vi "Sorting_Single_Frame_Displ_2.vi"(0 "(X,Y,dX,dY) IN":dbl[][](array[numeric]), 2 "error IN":errorcluster) -> (3 "Displ >1 Frame":dbl[][](array[numeric]), 4 "Displ =1 Frame":dbl[][](array[numeric]), 6 "error OUT":errorcluster)   [LabVIEW 2013]
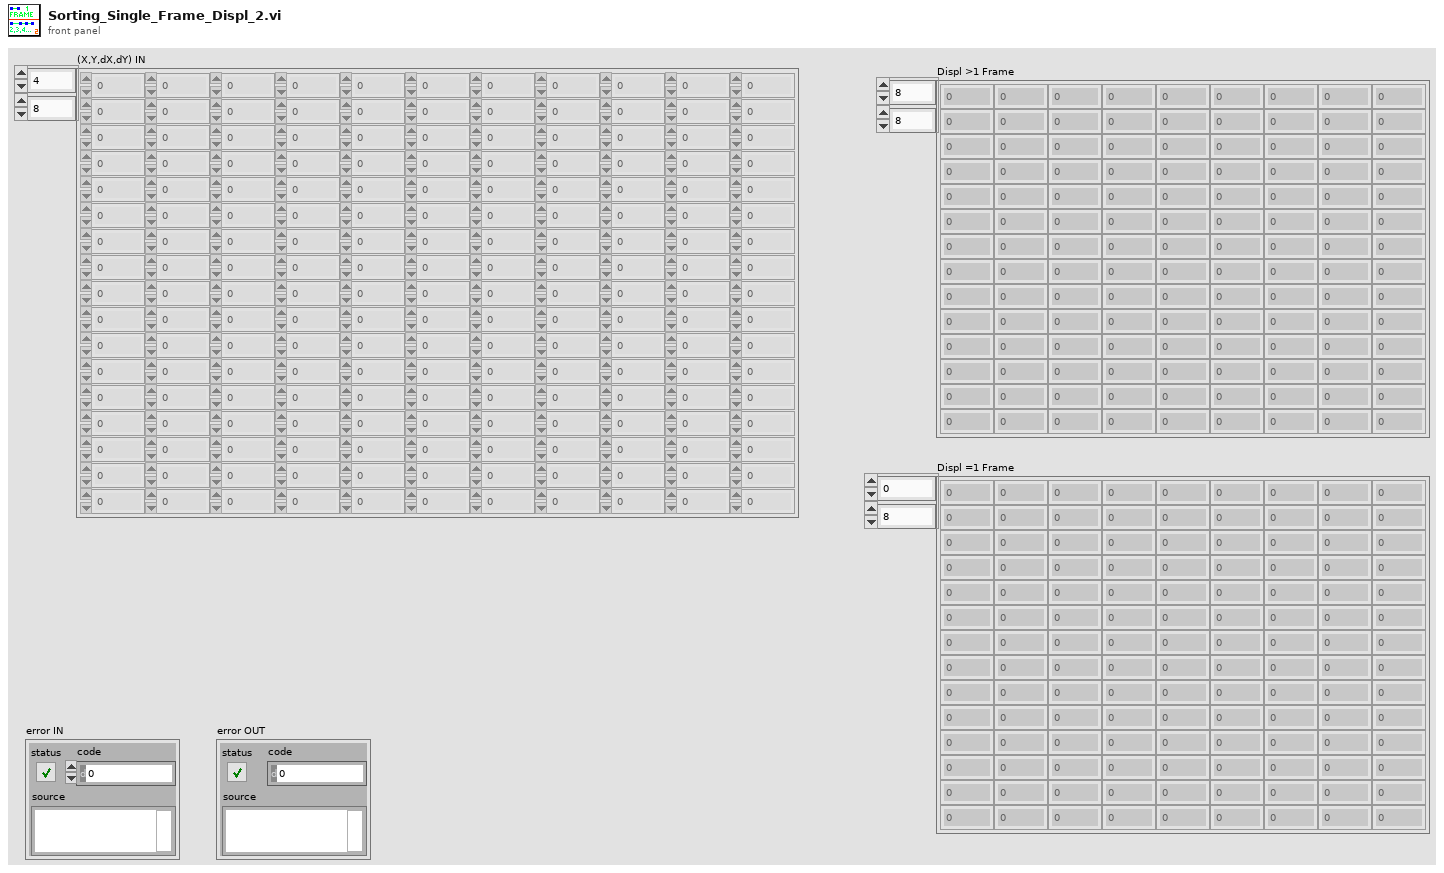
[diagram p1: front panel]
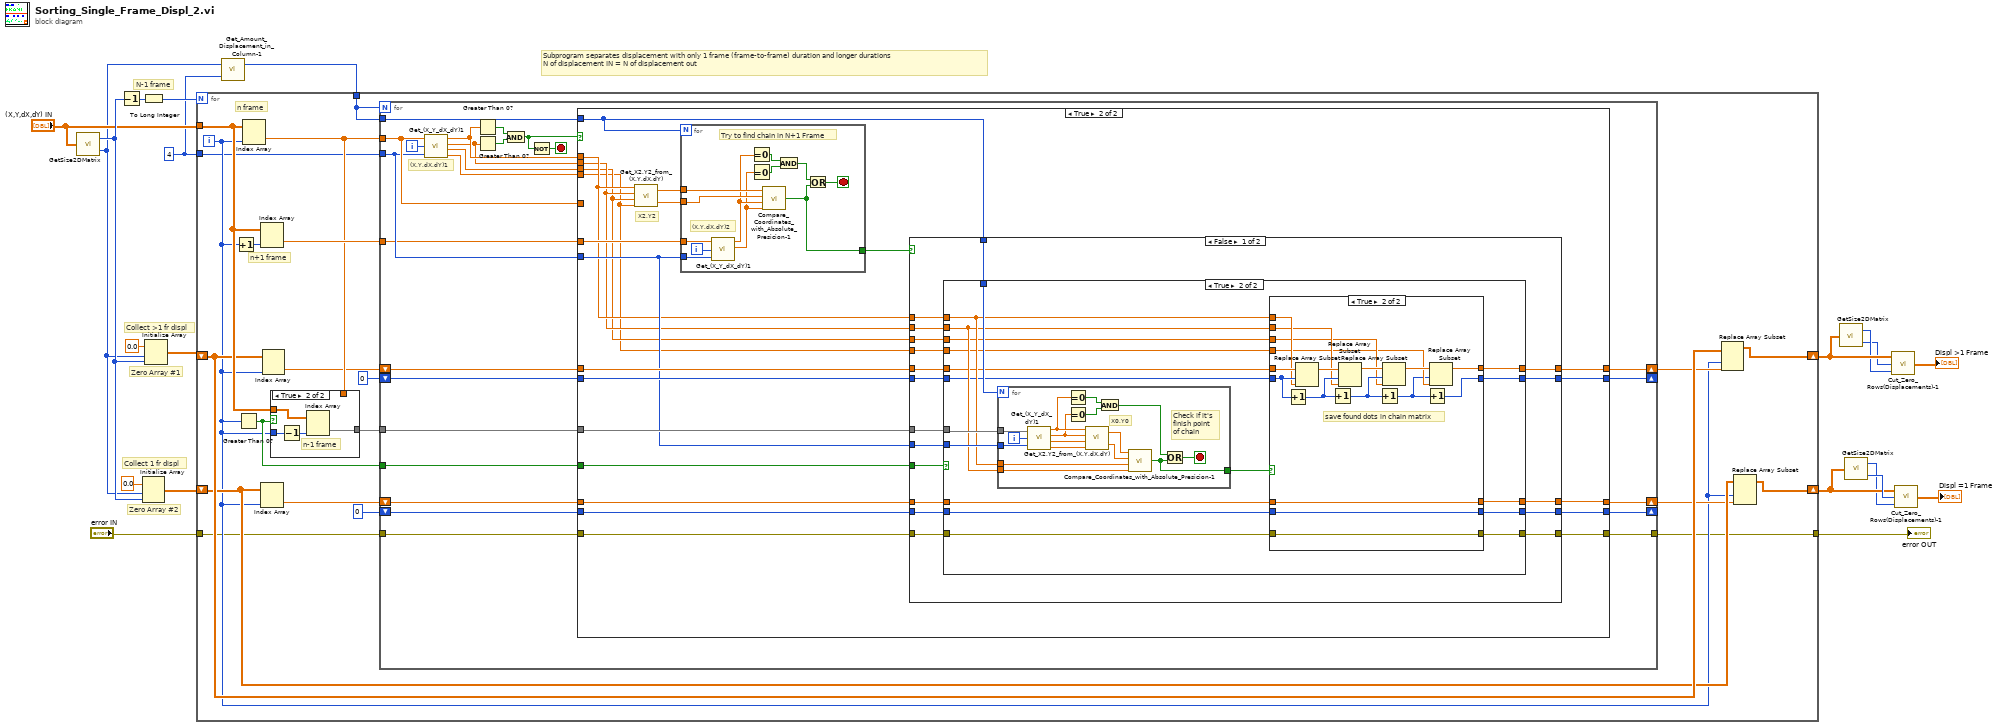
[diagram p0: block diagram]
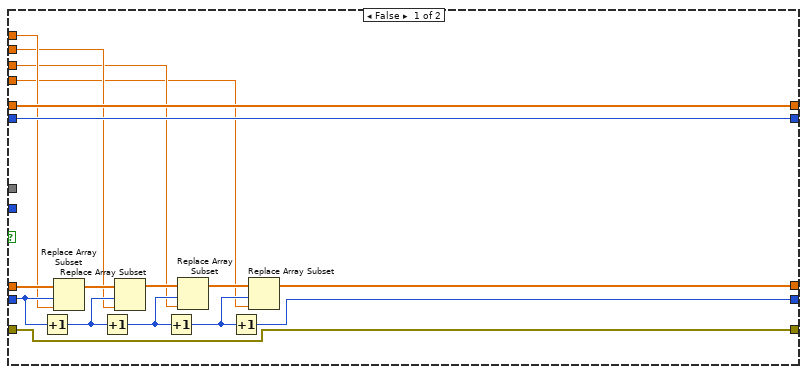
[diagram p4: hidden frame]
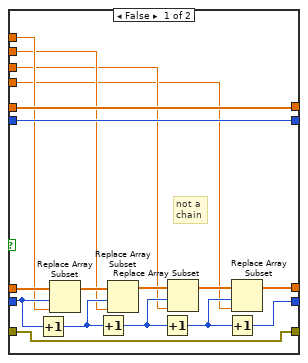
[diagram p5: hidden frame]
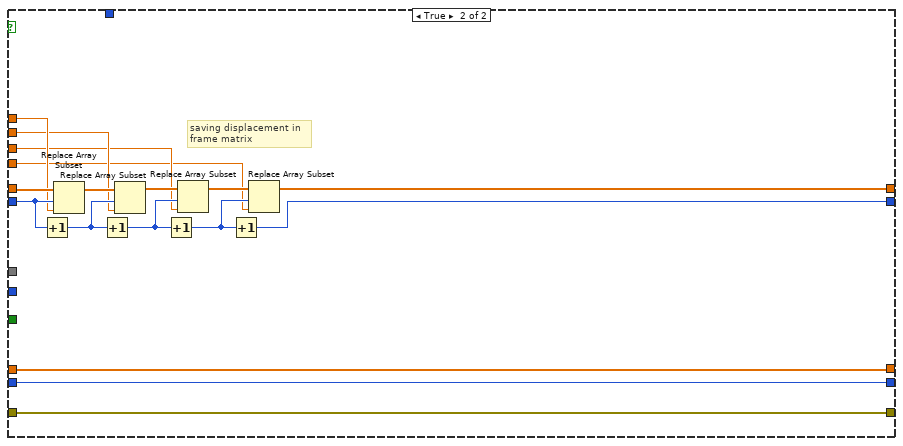
[diagram p6: hidden frame]
diagram:
  w2 = 4 ("y")
  # "Collect >1 fr displ"
  # "Collect 1 fr displ"
  # "Subprogram separates displacement with only 1 frame (frame-to-frame) duration and longer durations\nN of displacement IN = N of displacement out"
  # "Zero Array #2"
  # "Zero Array #1"
  # "N-1 frame"
  n1 = call "GetSize2DMatrix.vi"("Array IN (2D)"="(X,Y,dX,dY) IN") -> ("# Cols"=w16:i32, "# Rows"=w3:i32)
  n2 = Decrement(x=w16) -> (x-1=w21:i32)
  n3 = To Long Integer(number=w21) -> (32bit integer=w19:i32)
  n4 = Initialize Array(0.0 ("element"), w3, w16) -> (w15:dbl[][])
  n5 = Initialize Array(0.0 ("element"), w3, w16) -> (w18:dbl[][])
  n6 = call "Get_Amount_Displacement_in_Column-1.vi"("multiplier"=w2, "# Rows"=w3) -> ("Displ amount"=w1:i32)  [unwired: 1 out]
  n7 = for {
    N: w19 -> [_]
    shift-right: [w31] -> w13
    shift-left: w18 -> [w33]
    shift-right: [w27] -> w9
    shift-left: w15 -> [w29]
    tunnel: "(X,Y,dX,dY) IN" -> [w40]
    tunnel: "error IN" -> [w25]
    tunnel: [w24] -> w7
    tunnel: w2 -> [w23]
    tunnel: w1 -> [w22]
    i -> [w26]
    # "n+1 frame"
    # "n frame"
    n8 = Increment(x=w26) -> (x+1=w42:i32)
    n9 = Greater Than 0?(x=w26) -> (x > 0?=w37:bool)
    n10 = Index Array(array=w40, index (col)=w26) -> (element=w38:dbl[])  [unwired: 1 in]
    n11 = Index Array(array=w40, index (col)=w42) -> (element=w41:dbl[])  [unwired: 1 in]
    n12 = Index Array(array=w29, index (col)=w26) -> (element=w35:dbl[])  [unwired: 1 in]
    n13 = Index Array(array=w33, index (col)=w26) -> (element=w36:dbl[])  [unwired: 1 in]
    n14 = case shown="True" w37 {
      tunnel: w40 -> [_ w47]
      tunnel: w26 -> [_ w45]
      tunnel: [w43 w46] -> w39
      tunnel: w38 -> [w43 _]
      frame False {
      }
      frame True {
        # "n-1 frame"
        n15 = Decrement(x=w45) -> (x-1=w44:i32)
        n16 = Index Array(array=w47, index (col)=w44) -> (element=w46:dbl[])  [unwired: 1 in]
      }
    }
    n17 = for {
      N: w22 -> [_]
      tunnel: w41 -> [w62]
      tunnel: w23 -> [w67]
      tunnel: w22 -> [w69]
      tunnel: w38 -> [w68]
      tunnel: w39 -> [w54]
      tunnel: w37 -> [w59]
      shift-right: [w56] -> w32
      shift-left: w36 -> [w57]
      shift-right: [w50] -> w28
      shift-left: w35 -> [w53]
      shift-right: [w55] -> _
      shift-left: 0 -> [w58]
      shift-right: [w51] -> _
      shift-left: 0 -> [w52]
      tunnel: w25 -> [w49]
      tunnel: [w48] -> w24
      i -> [w72]
      stop <- w61 stop-if-true
      # "(X,Y,dX,dY)1"
      n18 = call "Get_(X_Y_dX_dY)1.vi"("(X,Y,dX,dY)"=w68, "index"=w72, "multiplier"=w67) -> ("X"=w66:dbl, "Y"=w65:dbl, "dX"=w64:dbl, "dY"=w63:dbl)
      n19 = Greater Than 0?(x=w66) -> (x > 0?=w71:bool)
      n20 = Greater Than 0?(x=w65) -> (x > 0?=w70:bool)
      n21 = And(x=w71, y=w70) -> (x .and. y?=w60:bool)
      n22 = Not(x=w60) -> (.not. x?=w61:bool)
      n23 = case shown="True" w60 {
        tunnel: w69 -> [_ w86]
        tunnel: w68 -> [_ _]
        tunnel: w67 -> [_ w87]
        tunnel: w66 -> [_ w83]
        tunnel: w65 -> [_ w80]
        tunnel: w64 -> [_ w79]
        tunnel: w63 -> [_ w78]
        tunnel: w62 -> [_ w99]
        tunnel: w59 -> [_ w95]
        tunnel: w58 -> [w76 w96]
        tunnel: w57 -> [w77 w97]
        tunnel: [w77 w90] -> w56
        tunnel: [w76 w89] -> w55
        tunnel: w54 -> [_ w88]
        tunnel: w53 -> [w75 w94]
        tunnel: w52 -> [w74 w93]
        tunnel: [w74 w91] -> w51
        tunnel: [w75 w92] -> w50
        tunnel: w49 -> [w73 w85]
        tunnel: [w73 w84] -> w48
        frame False {
        }
        frame True {
          # "X2,Y2"
          n24 = call "Get_X2,Y2_from_(X,Y,dX,dY).vi"("dY"=w78, "dX"=w79, "Y1"=w80, "X1"=w83) -> ("Y2 = (Y1+dY)"=w81:dbl, "X2 = (X1+dX)"=w82:dbl)
          n25 = for {
            N: w86 -> [_]
            tunnel: w82 -> [w224]
            tunnel: w81 -> [w223]
            tunnel: w99 -> [w231]
            tunnel: w87 -> [w228]
            tunnel: [w220] -> w98
            i -> [w227]
            stop <- w226 stop-if-true
            # "Try to find chain in N+1 Frame"
            # "(X,Y,dX,dY)2"
            n26 = call "Get_(X_Y_dX_dY)1.vi"("(X,Y,dX,dY)"=w231, "index"=w227, "multiplier"=w228) -> ("X"=w222:dbl, "Y"=w221:dbl)  [unwired: 2 out]
            n27 = Equal To 0?(x=w222) -> (x = 0?=w230:bool)
            n28 = Equal To 0?(x=w221) -> (x = 0?=w229:bool)
            n29 = call "Compare_Coordinates_with_Absolute_Presicion-1.vi"("X 1"=w224, "Y 1"=w223, "X 2"=w222, "Y 2"=w221) -> ("[OUT] Same coordinates?"=w220:bool)  [unwired: 1 in]
            n30 = And(x=w230, y=w229) -> (x .and. y?=w225:bool)
            n31 = Or(x=w225, y=w220) -> (x .or. y?=w226:bool)
          }
          n32 = case shown="False" w98 {
            tunnel: w83 -> [w111 w211]
            tunnel: w79 -> [w109 w209]
            tunnel: w80 -> [w110 w210]
            tunnel: w78 -> [w108 w208]
            tunnel: w97 -> [w116 w213]
            tunnel: w96 -> [w115 w212]
            tunnel: w95 -> [w117 _]
            tunnel: w94 -> [w114 w205]
            tunnel: w93 -> [w113 w204]
            tunnel: [w112 w205] -> w92
            tunnel: [w107 w204] -> w91
            tunnel: [w106 w207] -> w90
            tunnel: [w105 w206] -> w89
            tunnel: w88 -> [w104 _]
            tunnel: w87 -> [w103 _]
            tunnel: w86 -> [w102 _]
            tunnel: w85 -> [w101 w203]
            tunnel: [w100 w203] -> w84
            frame False {
              n33 = case shown="True" w117 {
                tunnel: w116 -> [w134 w144]
                tunnel: w115 -> [w133 w143]
                tunnel: [w134 w142] -> w106
                tunnel: [w133 w141] -> w105
                tunnel: w114 -> [w126 w140]
                tunnel: w113 -> [w125 w139]
                tunnel: [w124 w138] -> w112
                tunnel: w111 -> [w122 w148]
                tunnel: w110 -> [w121 w147]
                tunnel: w109 -> [w120 w146]
                tunnel: w108 -> [w119 w145]
                tunnel: [w123 w137] -> w107
                tunnel: w104 -> [_ w152]
                tunnel: w103 -> [_ w151]
                tunnel: w102 -> [_ w150]
                tunnel: w101 -> [w118 w136]
                tunnel: [w118 w135] -> w100
                frame False {
                  n34 = Increment(x=w125) -> (x+1=w131:i32)
                  n35 = Replace Array Subset(array=w126, new element=w122, index=w125) -> (w132:dbl[])
                  n36 = Increment(x=w131) -> (x+1=w128:i32)
                  n37 = Replace Array Subset(array=w132, new element=w121, index=w131) -> (w130:dbl[])
                  n38 = Increment(x=w128) -> (x+1=w127:i32)
                  n39 = Replace Array Subset(array=w130, new element=w120, index=w128) -> (w129:dbl[])
                  n40 = Increment(x=w127) -> (x+1=w123:i32)
                  n41 = Replace Array Subset(array=w129, new element=w119, index=w127) -> (w124:dbl[])
                }
                frame True {
                  n42 = for {
                    N: w150 -> [_]
                    tunnel: w152 -> [w202]
                    tunnel: w151 -> [w200]
                    tunnel: w148 -> [w189]
                    tunnel: w147 -> [w188]
                    tunnel: [w187] -> w149
                    i -> [w201]
                    stop <- w196 stop-if-true
                    # "Check if it's \nfinish point\nof chain"
                    # "X0,Y0"
                    n43 = call "Get_(X_Y_dX_dY)1.vi"("(X,Y,dX,dY)"=w202, "index"=w201, "multiplier"=w200) -> ("X"=w195:dbl, "Y"=w194:dbl, "dX"=w193:dbl, "dY"=w192:dbl)
                    n44 = Equal To 0?(x=w195) -> (x = 0?=w199:bool)
                    n45 = Equal To 0?(x=w194) -> (x = 0?=w198:bool)
                    n46 = call "Get_X2,Y2_from_(X,Y,dX,dY).vi"("dY"=w192, "dX"=w193, "Y1"=w194, "X1"=w195) -> ("Y2 = (Y1+dY)"=w190:dbl, "X2 = (X1+dX)"=w191:dbl)
                    n47 = And(x=w199, y=w198) -> (x .and. y?=w197:bool)
                    n48 = call "Compare_Coordinates_with_Absolute_Presicion-1.vi"("X 1"=w191, "Y 1"=w190, "X 2"=w189, "Y 2"=w188) -> ("[OUT] Same coordinates?"=w187:bool)  [unwired: 1 in]
                    n49 = Or(x=w197, y=w187) -> (x .or. y?=w196:bool)
                  }
                  n50 = case shown="True" w149 {
                    tunnel: w148 -> [w159 w177]
                    tunnel: w147 -> [w158 w176]
                    tunnel: w146 -> [w157 w175]
                    tunnel: w145 -> [w156 w174]
                    tunnel: w144 -> [w169 w181]
                    tunnel: w143 -> [w168 w180]
                    tunnel: [w169 w179] -> w142
                    tunnel: [w168 w178] -> w141
                    tunnel: w140 -> [w161 w172]
                    tunnel: w139 -> [w160 w171]
                    tunnel: [w155 w172] -> w138
                    tunnel: [w154 w171] -> w137
                    tunnel: w136 -> [w153 w170]
                    tunnel: [w153 w170] -> w135
                    frame False {
                      # "not a \nchain"
                      n51 = Increment(x=w160) -> (x+1=w166:i32)
                      n52 = Replace Array Subset(array=w161, new element=w159, index=w160) -> (w167:dbl[])
                      n53 = Increment(x=w166) -> (x+1=w163:i32)
                      n54 = Replace Array Subset(array=w167, new element=w158, index=w166) -> (w165:dbl[])
                      n55 = Increment(x=w163) -> (x+1=w162:i32)
                      n56 = Replace Array Subset(array=w165, new element=w157, index=w163) -> (w164:dbl[])
                      n57 = Increment(x=w162) -> (x+1=w154:i32)
                      n58 = Replace Array Subset(array=w164, new element=w156, index=w162) -> (w155:dbl[])
                    }
                    frame True {
                      # "save found dots in chain matrix"
                      n59 = Increment(x=w180) -> (x+1=w185:i32)
                      n60 = Replace Array Subset(array=w181, new element=w177, index=w180) -> (w186:dbl[])
                      n61 = Increment(x=w185) -> (x+1=w182:i32)
                      n62 = Replace Array Subset(array=w186, new element=w176, index=w185) -> (w184:dbl[])
                      n63 = Increment(x=w182) -> (x+1=w173:i32)
                      n64 = Replace Array Subset(array=w184, new element=w175, index=w182) -> (w183:dbl[])
                      n65 = Increment(x=w173) -> (x+1=w178:i32)
                      n66 = Replace Array Subset(array=w183, new element=w174, index=w173) -> (w179:dbl[])
                    }
                  }
                }
              }
            }
            frame True {
              # "saving displacement in \nframe matrix"
              n67 = Increment(x=w212) -> (x+1=w218:i32)
              n68 = Replace Array Subset(array=w213, new element=w211, index=w212) -> (w219:dbl[])
              n69 = Increment(x=w218) -> (x+1=w215:i32)
              n70 = Replace Array Subset(array=w219, new element=w210, index=w218) -> (w217:dbl[])
              n71 = Increment(x=w215) -> (x+1=w214:i32)
              n72 = Replace Array Subset(array=w217, new element=w209, index=w215) -> (w216:dbl[])
              n73 = Increment(x=w214) -> (x+1=w206:i32)
              n74 = Replace Array Subset(array=w216, new element=w208, index=w214) -> (w207:dbl[])
            }
          }
        }
      }
    }
    n75 = Replace Array Subset(array=w33, new element=w32, index (col)=w26) -> (w31:dbl[][])  [unwired: 1 in]
    n76 = Replace Array Subset(array=w29, new element=w28, index (col)=w26) -> (w27:dbl[][])  [unwired: 1 in]
  }
  "error OUT" <- w7
  n77 = call "GetSize2DMatrix.vi"("Array IN (2D)"=w13) -> ("# Cols"=w12:i32, "# Rows"=w11:i32)
  n78 = call "GetSize2DMatrix.vi"("Array IN (2D)"=w9) -> ("# Cols"=w8:i32, "# Rows"=w10:i32)
  n79 = call "Cut_Zero_Rows(Displacements)-1.vi"("# Cols"=w12, "# Rows"=w11, "Array IN"=w13) -> ("Array OUT"=→"Displ >1 Frame":dbl[][])
  n80 = call "Cut_Zero_Rows(Displacements)-1.vi"("# Cols"=w8, "# Rows"=w10, "Array IN"=w9) -> ("Array OUT"=→"Displ =1 Frame":dbl[][])
